vi "ReadLogFileFromDisk.vi"(8 "error in (no error)":errorcluster, 11 "Log File path":path) -> (0 "error out":errorcluster, 3 "Messages":T1)   [LabVIEW 2011]
uses:
  LogFileData.ctl
  030 - EVENTS/03 - ToMessageHandlerProcess/ToMessageHandlerEvent.ctl
  030 - EVENTS/03 - ToMessageHandlerProcess/enumMessageCriticity.ctl
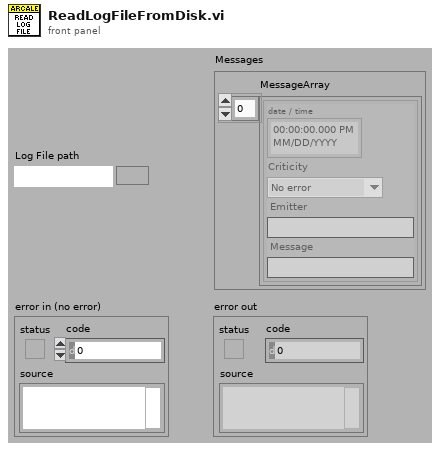
[diagram p1: front panel]
types:
  T1 = typedef "LogFileData.ctl" = cluster{"MessageArray":T2[]}
  T2 = typedef "ToMessageHandlerEvent.ctl" = cluster{"date / time":timestamp, "Criticity":T3, "Emitter":string, "Message":string}
  T3 = typedef "enumMessageCriticity.ctl" = enum16{"No error", "Info", "Warning", "Error", "Fatal error"}
  T4 = enum16{"open", "replace", "create", "open or create", "replace or create", "replace or create with confirmation"}
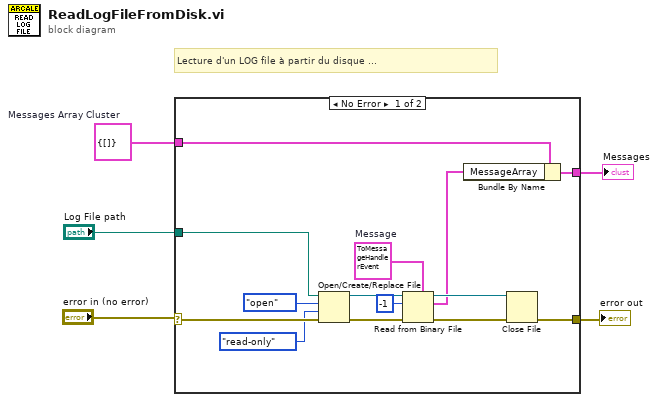
[diagram p0: block diagram]
diagram:
  w1 = T1 {"MessageArray"=[]}  # Messages Array Cluster
  # "Lecture d'un LOG file à partir du disque ..."
  n1 = case shown="No Error" "error in (no error)" {
    selector: "error in (no error)" -> [w19 w21]
    tunnel: [w11 w21] -> w4
    tunnel: "Log File path" -> [w18 _]
    tunnel: [w8 w20] -> w2
    tunnel: w1 -> [w7 w20]
    frame No Error {
      w6 = T2 {"date / time"=timestamp(0 s since 1904-01-01), "Criticity"=enum."No error", "Emitter"="", "Message"=""}  # Message
      n2 = Open/Create/Replace File(file path (use dialog)=w18, error in=w19, operation (0:open)=T4."open", access (0:read/write)=enum16{"read/write", "read-only", "write-only"}."read-only") -> (refnum out=w15:refnum<file>, error out=w14:errorcluster)  [unwired: 2 in, 1 out]
      n3 = Read from Binary File(5:w6, 8:w14, 10:-1 ("count (1)"), 11:w15) -> (0:w13:errorcluster, 2:w9:T2[], 3:w12:refnum<file>)  [unwired: 2 in, 1 out]
      n4 = Bundle By Name(cluster=w7, "MessageArray"=w9) -> (w8:T1)
      n5 = Close File(refnum=w12, error in=w13) -> (error out=w11:errorcluster)  [unwired: 1 out]
    }
    frame Error {
    }
  }
  "error out" <- w4
  "Messages" <- w2
